vi "PCandDVR.vi"() -> ()   [LabVIEW 2013]
doc: "Use this template to build a producer/consumer design pattern with events to produce queue items. Use this design pattern instead of the User Interface Event Handler pattern for user interfaces when you want to execute code asynchronously in response to an event without slowing the user interface responsiveness."
uses:
  Control/SignalType.ctl
  Control/SystemCommand.ctl
  Control/SubDaqCommand.ctl
panel:
  out "FFT":cluster{"f0":dbl, "df":dbl, "magnitude":dbl[]}[](graph)
  out "State":string
  in  "SignalType":T1
  in  "Stop":bool
  in  "Start":bool
  in  "Amplitude":dbl=1.0
  in  "Frequency":dbl=100.0
  out "Waveform":waveform(dbl)[](graph)
  out "Numeric Ind":dbl
  out "Boolean Ind":bool
  out "String Ind":string
  in  "InvertBool":bool
  in  "SquareNumeric":bool
  in  "ReverseString":bool
  in  "Numeric":dbl
  in  "Boolean":bool
  in  "String":string
  in  "ReadValueInProducer":bool
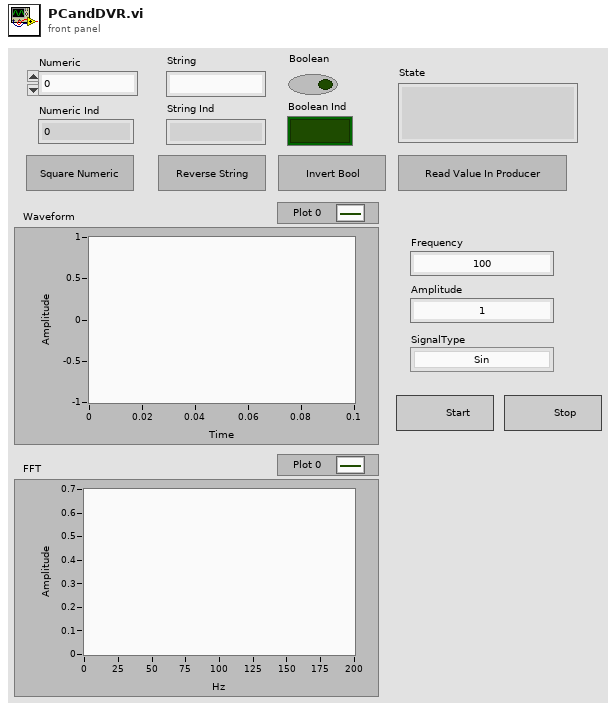
[diagram p1: front panel]
types:
  T1 = typedef "SignalType.ctl" = enum16{"Sin", "Triangle", "Square"}
  T2 = cluster{"DVReference out":refnum<data-value>, "MainQueueOut":refnum<queue>, "SubQueueOut":refnum<queue>}
  T3 = typedef "SystemCommand.ctl" = enum16{"None", "Init", "Close", "ShowNumeric", "ShowString", "ShowBool", "SquareNumeric", "ReverseString", "InvertBool", "FFT"}
  T4 = typedef "SystemData.ctl" = cluster{"Numeric":dbl, "String":string, "Boolean":bool, "Frequency":dbl, "Amplitude":dbl, "SignalType":T1, "WaveformArray":waveform(dbl)[], "Reset":bool, "StateString":string, "FFTmagnitudes":cluster{"f0":dbl, "df":dbl, "magnitude":dbl[]}[]}
  T5 = typedef "SubDaqCommand.ctl" = enum16{"None", "Init", "Work", "Stop", "Close"}
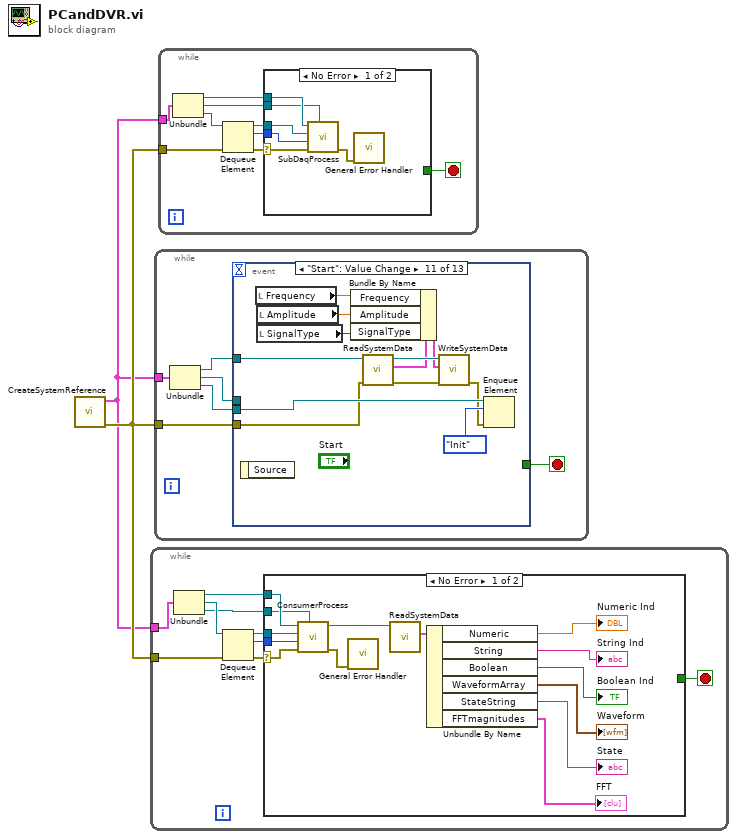
[diagram p0: block diagram]
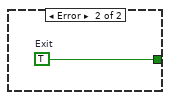
[diagram p2: hidden frame]
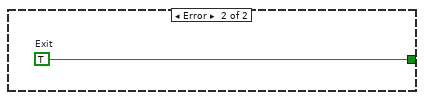
[diagram p3: hidden frame]
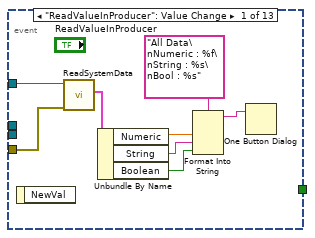
[diagram p4: hidden frame]
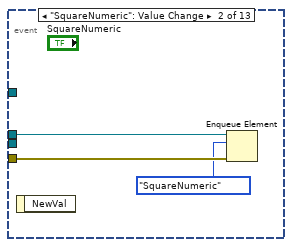
[diagram p5: hidden frame]
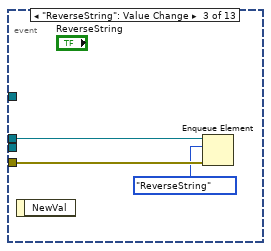
[diagram p6: hidden frame]
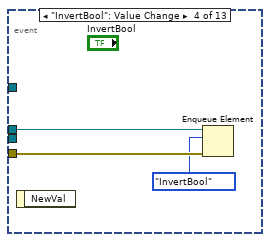
[diagram p7: hidden frame]
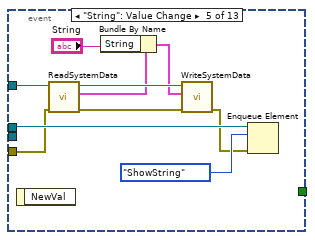
[diagram p8: hidden frame]
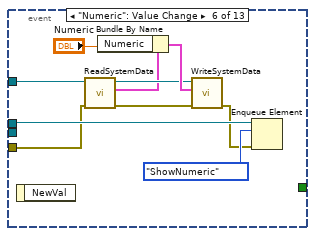
[diagram p9: hidden frame]
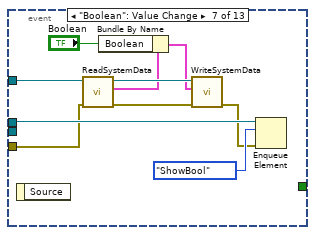
[diagram p10: hidden frame]
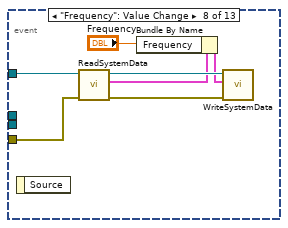
[diagram p11: hidden frame]
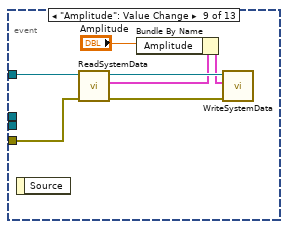
[diagram p12: hidden frame]
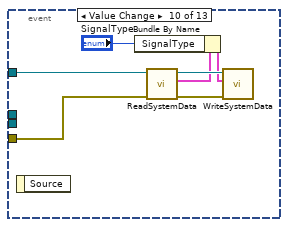
[diagram p13: hidden frame]
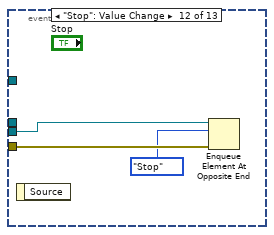
[diagram p14: hidden frame]
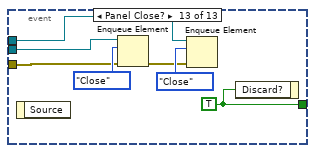
[diagram p15: hidden frame]
diagram:
  n1 = call "CreateSystemReference.vi"() -> ("error out"=w2:errorcluster, "Cluster"=w1:T2)  [unwired: 10 in]
  n2 = while {
    tunnel: w2 -> [w7]
    tunnel: w1 -> [w6]
    stop <- w9 stop-if-true
    n3 = Unbundle(w6) -> ("DVReference out"=w5:refnum<data-value>, "MainQueueOut"=w4:refnum<queue>, "SubQueueOut"=w3:refnum<queue>)
    n4 = Dequeue Element(queue=w4, error in (no error)=w7) -> (queue out=w8:refnum<queue>, element=w10:T3, error out=w11:errorcluster)  [unwired: 1 in, 1 out]
    n5 = case shown="No Error" w11 {
      selector: w11 -> [w24 _]
      tunnel: w10 -> [w25 _]
      tunnel: [_ w26] -> w9
      tunnel: w5 -> [w18 _]
      tunnel: w8 -> [w23 _]
      tunnel: w3 -> [w15 _]
      frame No Error {
        n6 = call "ConsumerProcess.vi"("SubQueueIN"=w15, "error in (no error)"=w24, "Command"=w25, "MainQueueIN"=w23, "Data Value Reference IN"=w18) -> ("error out"=w19:errorcluster, "Data Value Reference out"=w17:refnum<data-value>)  [unwired: 5 in]
        n7 = call <vilib>:"General Error Handler.vi"("error in (no error)"=w19) -> ()  [unwired: 10 in, 5 out]
        n8 = call "ReadSystemData.vi"("Data Value Reference IN"=w17) -> ("SystemDataCluster"=w16:T4)  [unwired: 8 in, 2 out]
        n9 = Unbundle By Name(w16) -> ("Numeric"=→"Numeric Ind":dbl, "String"=→"String Ind":string, "Boolean"=→"Boolean Ind":bool, "WaveformArray"=→"Waveform":waveform(dbl)[], "StateString"=→"State":string, "FFTmagnitudes"=→"FFT":cluster{"f0":dbl, "df":dbl, "magnitude":dbl[]}[])
      }
      frame Error {
        w26 = TRUE  # Exit
      }
    }
  }
  n10 = while {
    tunnel: w2 -> [w32]
    tunnel: w1 -> [w30]
    stop <- w31 stop-if-true
    n11 = Unbundle(w30) -> ("DVReference out"=w29:refnum<data-value>, "MainQueueOut"=w28:refnum<queue>, "SubQueueOut"=w27:refnum<queue>)
    n12 = event shown="[10] \"Start\": Value Change" {
      selector: _ -> [_ _ _ _ _ _ _ _ _ _ _ _ _]
      dyn-events: _ -> [_ _ _ _ _ _ _ _ _ _ _ _ _]
      timeout: _ -> [_ _ _ _ _ _ _ _ _ _ _ _ _]
      tunnel: w28 -> [_ w43 w46 w49 w59 w69 w79 _ _ _ _ _ w121]
      tunnel: w32 -> [w39 w42 w45 w48 w52 w61 w73 w84 w91 w98 w106 w115 w117]
      tunnel: [_ _ _ _ _ _ _ _ _ _ _ _ w122] -> w31
      tunnel: w29 -> [w40 _ _ _ w56 w66 w77 w86 w93 w100 w101 _ _]
      tunnel: w27 -> [_ _ _ _ _ _ _ _ _ _ w112 w114 w116]
      event "ReadValueInProducer": Value Change {
        n13 = event-data() -> ()  [unwired: 1 in, 1 out]
        n14 = call "ReadSystemData.vi"("error in (no error)"=w39, "Data Value Reference IN"=w40) -> ("SystemDataCluster"=w33:T4)  [unwired: 7 in, 2 out]
        n15 = Unbundle By Name(w33) -> ("Numeric"=w36:dbl, "String"=w35:string, "Boolean"=w34:bool)
        n16 = Format Into String(format string="All Data\nNumeric : %f\nString : %s\nBool : %s", w36, w35, w34) -> (resulting string=w37:string)  [unwired: 2 in, 1 out]
        n17 = One Button Dialog(message=w37) -> ()  [unwired: 1 in, 1 out]
      }
      event "SquareNumeric": Value Change {
        n18 = event-data() -> ()  [unwired: 1 in, 1 out]
        n19 = Enqueue Element(queue=w43, element=SystemCommand."SquareNumeric" ("Command"), error in (no error)=w42) -> ()  [unwired: 1 in, 3 out]
      }
      event "ReverseString": Value Change {
        n20 = event-data() -> ()  [unwired: 1 in, 1 out]
        n21 = Enqueue Element(queue=w46, element=SystemCommand."ReverseString" ("Command"), error in (no error)=w45) -> ()  [unwired: 1 in, 3 out]
      }
      event "InvertBool": Value Change {
        n22 = event-data() -> ()  [unwired: 1 in, 1 out]
        n23 = Enqueue Element(queue=w49, element=SystemCommand."InvertBool" ("Command"), error in (no error)=w48) -> ()  [unwired: 1 in, 3 out]
      }
      event "String": Value Change {
        n24 = event-data() -> ()  [unwired: 1 in, 1 out]
        n25 = call "ReadSystemData.vi"("error in (no error)"=w52, "Data Value Reference IN"=w56) -> ("error out"=w53:errorcluster, "SystemDataCluster"=w51:T4, "Data Value Reference out"=w54:refnum<data-value>)  [unwired: 7 in]
        n26 = Bundle By Name(cluster=w51, "String"="String") -> (w50:T4)
        n27 = call "WriteSystemData.vi"("error in (no error)"=w53, "SystemDataCluster"=w50, "Data Value Reference IN"=w54) -> ("error out"=w55:errorcluster)  [unwired: 7 in, 1 out]
        n28 = Enqueue Element(queue=w59, element=SystemCommand."ShowString" ("Command"), error in (no error)=w55) -> ()  [unwired: 1 in, 3 out]
      }
      event "Numeric": Value Change {
        n29 = event-data() -> ()  [unwired: 1 in, 1 out]
        n30 = call "ReadSystemData.vi"("error in (no error)"=w61, "Data Value Reference IN"=w66) -> ("error out"=w62:errorcluster, "SystemDataCluster"=w60:T4, "Data Value Reference out"=w63:refnum<data-value>)  [unwired: 7 in]
        n31 = Bundle By Name(cluster=w60, "Numeric"="Numeric") -> (w64:T4)
        n32 = call "WriteSystemData.vi"("error in (no error)"=w62, "SystemDataCluster"=w64, "Data Value Reference IN"=w63) -> ("error out"=w65:errorcluster)  [unwired: 7 in, 1 out]
        n33 = Enqueue Element(queue=w69, element=SystemCommand."ShowNumeric" ("Command"), error in (no error)=w65) -> ()  [unwired: 1 in, 3 out]
      }
      event "Boolean": Value Change {
        n34 = event-data() -> ()  [unwired: 1 in, 1 out]
        n35 = call "ReadSystemData.vi"("error in (no error)"=w73, "Data Value Reference IN"=w77) -> ("error out"=w72:errorcluster, "SystemDataCluster"=w71:T4, "Data Value Reference out"=w74:refnum<data-value>)  [unwired: 7 in]
        n36 = Bundle By Name(cluster=w71, "Boolean"="Boolean") -> (w70:T4)
        n37 = call "WriteSystemData.vi"("error in (no error)"=w72, "SystemDataCluster"=w70, "Data Value Reference IN"=w74) -> ("error out"=w76:errorcluster)  [unwired: 7 in, 1 out]
        n38 = Enqueue Element(queue=w79, element=SystemCommand."ShowBool" ("Command"), error in (no error)=w76) -> ()  [unwired: 1 in, 3 out]
      }
      event "Frequency": Value Change {
        n39 = event-data() -> ()  [unwired: 1 in, 1 out]
        n40 = call "ReadSystemData.vi"("error in (no error)"=w84, "Data Value Reference IN"=w86) -> ("error out"=w83:errorcluster, "SystemDataCluster"=w82:T4, "Data Value Reference out"=w85:refnum<data-value>)  [unwired: 7 in]
        n41 = Bundle By Name(cluster=w82, "Frequency"="Frequency") -> (w81:T4)
        n42 = call "WriteSystemData.vi"("error in (no error)"=w83, "SystemDataCluster"=w81, "Data Value Reference IN"=w85) -> ()  [unwired: 7 in, 2 out]
      }
      event "Amplitude": Value Change {
        n43 = event-data() -> ()  [unwired: 1 in, 1 out]
        n44 = call "ReadSystemData.vi"("error in (no error)"=w91, "Data Value Reference IN"=w93) -> ("error out"=w90:errorcluster, "SystemDataCluster"=w89:T4, "Data Value Reference out"=w92:refnum<data-value>)  [unwired: 7 in]
        n45 = Bundle By Name(cluster=w89, "Amplitude"="Amplitude") -> (w88:T4)
        n46 = call "WriteSystemData.vi"("error in (no error)"=w90, "SystemDataCluster"=w88, "Data Value Reference IN"=w92) -> ()  [unwired: 7 in, 2 out]
      }
      event Value Change {
        n47 = event-data() -> ()  [unwired: 1 in, 1 out]
        n48 = call "ReadSystemData.vi"("error in (no error)"=w98, "Data Value Reference IN"=w100) -> ("error out"=w97:errorcluster, "SystemDataCluster"=w96:T4, "Data Value Reference out"=w99:refnum<data-value>)  [unwired: 7 in]
        n49 = Bundle By Name(cluster=w96, "SignalType"="SignalType") -> (w95:T4)
        n50 = call "WriteSystemData.vi"("error in (no error)"=w97, "SystemDataCluster"=w95, "Data Value Reference IN"=w99) -> ()  [unwired: 7 in, 2 out]
      }
      event "Start": Value Change {
        n51 = event-data() -> ()  [unwired: 1 in, 1 out]
        n52 = local read "Frequency"() -> (w102:dbl)
        n53 = local read "Amplitude"() -> (w103:dbl)
        n54 = local read "SignalType"() -> (w104:T1)
        n55 = call "ReadSystemData.vi"("error in (no error)"=w106, "Data Value Reference IN"=w101) -> ("error out"=w109:errorcluster, "SystemDataCluster"=w108:T4, "Data Value Reference out"=w110:refnum<data-value>)  [unwired: 7 in]
        n56 = Bundle By Name(cluster=w108, "Frequency"=w102, "Amplitude"=w103, "SignalType"=w104) -> (w107:T4)
        n57 = call "WriteSystemData.vi"("error in (no error)"=w109, "SystemDataCluster"=w107, "Data Value Reference IN"=w110) -> ("error out"=w105:errorcluster)  [unwired: 7 in, 1 out]
        n58 = Enqueue Element(queue=w112, element=SubDaqCommand."Init" ("SubDaqCommand"), error in (no error)=w105) -> ()  [unwired: 1 in, 3 out]
      }
      event "Stop": Value Change {
        n59 = event-data() -> ()  [unwired: 1 in, 1 out]
        n60 = Enqueue Element At Opposite End(queue=w114, element=SubDaqCommand."Stop" ("SubDaqCommand"), error in (no error)=w115) -> ()  [unwired: 1 in, 3 out]
      }
      event Panel Close? {
        w122 = TRUE ("stop")
        n61 = event-data() -> ()  [unwired: 1 in, 1 out]
        n62 = Enqueue Element(queue=w116, element=SubDaqCommand."Close", error in (no error)=w117) -> (error out=w118:errorcluster)  [unwired: 1 in, 2 out]
        n63 = Enqueue Element(queue=w121, element=SystemCommand."Close" ("Command"), error in (no error)=w118) -> ()  [unwired: 1 in, 3 out]
        n64 = event-data("Discard?"=w122) -> ()  [unwired: 1 in, 1 out]
      }
    }
  }
  n65 = while {
    tunnel: w2 -> [w127]
    tunnel: w1 -> [w126]
    stop <- w129 stop-if-true
    n66 = Unbundle(w126) -> ("DVReference out"=w123:refnum<data-value>, "MainQueueOut"=w124:refnum<queue>, "SubQueueOut"=w125:refnum<queue>)
    n67 = Dequeue Element(queue=w125, error in (no error)=w127) -> (queue out=w128:refnum<queue>, element=w130:T5, error out=w131:errorcluster)  [unwired: 1 in, 1 out]
    n68 = case shown="No Error" w131 {
      selector: w131 -> [w134 _]
      tunnel: w130 -> [w132 _]
      tunnel: [_ w138] -> w129
      tunnel: w128 -> [w137 _]
      tunnel: w124 -> [w135 _]
      tunnel: w123 -> [w136 _]
      frame No Error {
        n69 = call "SubDaqProcess.vi"("MainQueueIN"=w135, "error in (no error)"=w134, "SubDaqCommand"=w132, "SubQueueIN"=w137, "Data Value Reference IN"=w136) -> ("error out"=w133:errorcluster)  [unwired: 5 in, 1 out]
        n70 = call <vilib>:"General Error Handler.vi"("error in (no error)"=w133) -> ()  [unwired: 10 in, 5 out]
      }
      frame Error {
        w138 = TRUE  # Exit
      }
    }
  }
